vi "Store Channel State.vi"(8 "error in (no error)":errorcluster, 10 "Memory Register (0: A)":u16(ring) items=["A", "B", "C", "D"], 11 "VISA resource name":refnum<visa-resource-name>) -> (0 "error out":errorcluster, 3 "VISA resource name out":refnum<visa-resource-name>)   [LabVIEW 2020, in "Agilent ENA Series.lvlib"]
doc: "Saves the instrument state of the items set for the active channel specific to that channel only into the specified register (volatile memory).\n\nNotes:\nNotice that, if an instrument state has been saved already in the specified register, its contents are overwritten."
uses:
  <instrlib>/Agilent ENA Series/Agilent ENA Series.lvlib
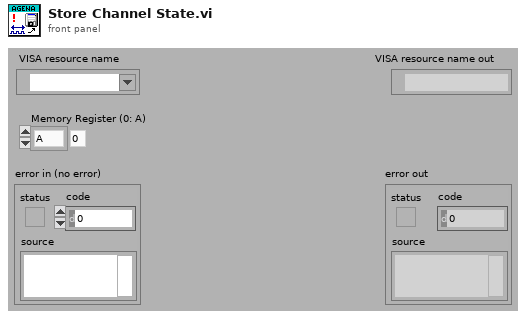
[diagram p1: front panel]
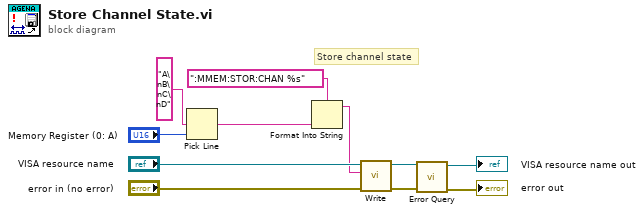
[diagram p0: block diagram]
diagram:
  # "Store channel state"
  n1 = Pick Line(multi-line string="A\nB\nC\nD", line index="Memory Register (0: A)") -> (output string=w5:string)  [unwired: 1 in]
  n2 = Format Into String(format string=":MMEM:STOR:CHAN %s", w5) -> (resulting string=w8:string)  [unwired: 2 in, 1 out]
  n3 = call <instrlib>:"Write.vi"("error in (no error)"="error in (no error)", "String ()"=w8, "VISA resource name"="VISA resource name") -> ("error out"=w3:errorcluster, "VISA resource name out"=w4:refnum<visa-resource-name>)  [unwired: 6 in, 1 out]
  n4 = call <instrlib>:"Error Query.vi"("error in (no error)"=w3, "VISA resource name"=w4) -> ("error out"=→"error out":errorcluster, "VISA resource name out"=→"VISA resource name out":refnum<visa-resource-name>)  [unwired: 6 in, 2 out]
